vi "Actor Core.vi"(8 "error in":errorcluster, 11 "RandomDataChart in":refnum<class "ValueInputs.lvclass">) -> (0 "error out":errorcluster, 3 "Actor out":refnum<class "Actor.lvclass">)   [LabVIEW 2015, in "TestViewables.lvlib" / "ValueInputs.lvclass"]
doc: "(<B>Filename</B>: Actor Framework.lvlib:Actor.lvclass:Actor Core.vi)\n\nReceives messages to the actor, reacts to them, and initiates any error handling that may shut the actor down.\n\nDescendant classes may override this VI to append parallel tasks for the actor to complete while it handles messages. Overrides use the Call Parent Method node.\n\n<License>\nCopyright © 2017 Composed Systems, LLC | All rights reserved\nwww.composed.io\n\nAuthor: Ethan Stern <ethan.stern@composed.io>\n\nThis software is provided \"AS IS\" WITHOUT WARRANTIES, either express or implied, AND IS FOR EDUCATIONAL PURPOSES ONLY.\n</License>"
uses:
  ValueInputs.lvclass
  <vilib>/ActorFramework/Actor/Actor.lvclass
  <vilib>/ActorFramework/Actor/Actor.lvclass/Actor.ctl
  <vilib>/ActorFramework/Message Enqueuer/Message Enqueuer.lvclass/Message Enqueuer.ctl
  <vilib>/ActorFramework/Message Enqueuer/Init from Existing Queue.vi
  Framework/IViewable/IViewable/IViewable.lvclass
  <vilib>/ActorFramework/Message Enqueuer/Message Enqueuer.lvclass
  Framework/AutoRegistration/ActorAutoRegistration Messages/ValueChangeMsg/ValueChangeMsg.lvclass
panel:
  in  "ID":i32
  in  "Flavor":string
  in  "Setpoint":dbl
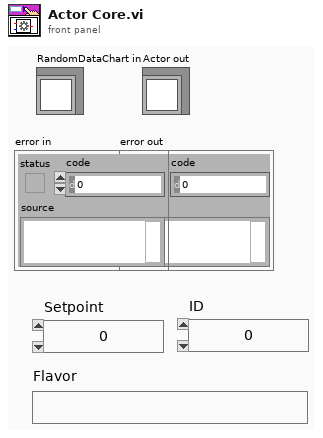
[diagram p1: front panel]
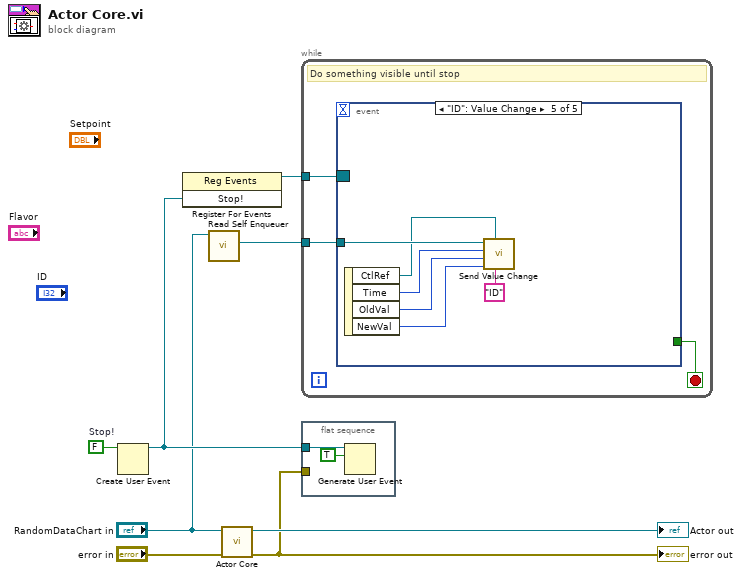
[diagram p0: block diagram]
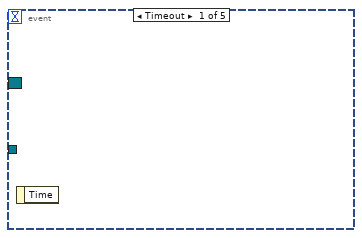
[diagram p2: hidden frame]
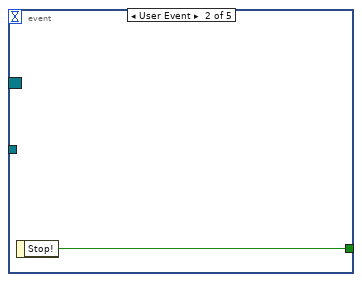
[diagram p3: hidden frame]
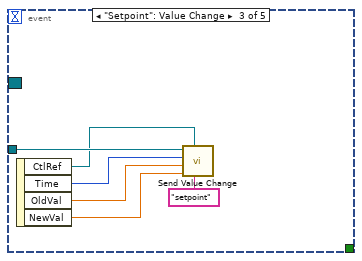
[diagram p4: hidden frame]
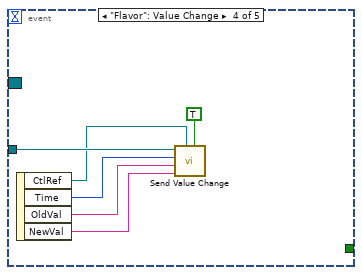
[diagram p5: hidden frame]
diagram:
  w6 = FALSE  # Stop!
  n1 = Create User Event(user event datatype=w6) -> (user event=w3:refnum<user-event>)  [unwired: 1 in, 1 out]
  n2 = register-events(w3) -> (reference out=w4:refnum<event-registration>)  [unwired: 2 in, 1 out]
  n3 = call <vilib>:"Read Self Enqueuer.vi"("Actor"="RandomDataChart in") -> ("Self Enqueuer"=w1:refnum<class "Message Enqueuer.lvclass">)  [unwired: 10 in]
  n4 = call-parent "Actor Core.vi"("error in"="error in", "IViewable In"="RandomDataChart in") -> ("error out"=w5:errorcluster, "Actor out"=→"Actor out":refnum<class "Actor.lvclass">)  [unwired: 8 in]
  "error out" <- w5
  n5 = while {
    tunnel: w4 -> [w11]
    tunnel: w1 -> [w9]
    stop <- w10 stop-if-true
    # "Do something visible until stop"
    n6 = event shown="[4] \"ID\": Value Change" {
      selector: w11 -> [_ _ _ _ _]
      dyn-events: _ -> [_ _ _ _ _]
      timeout: _ -> [_ _ _ _ _]
      tunnel: [_ w12 _ _ _] -> w10
      tunnel: w9 -> [_ _ w18 w24 w30]
      event Timeout {
        n7 = event-data() -> ()  [unwired: 1 in, 1 out]
      }
      event User Event {
        n8 = event-data() -> ("Stop!"=w12:bool)  [unwired: 1 in]
      }
      event "Setpoint": Value Change {
        n9 = event-data() -> ("CtlRef"=w13:refnum<vi>, "Time"=w14:u32, "OldVal"=w17:dbl, "NewVal"=w15:dbl)  [unwired: 1 in]
        n10 = call "Send Value Change.vi"("Name (Get Text From Control)"="setpoint" ("Name"), "Ctl Refnum"=w13, "New Value"=w15, "Old Value"=w17, "Time"=w14, "Message Enqueuer in"=w18) -> ()  [unwired: 5 in, 1 out]
      }
      event "Flavor": Value Change {
        n11 = event-data() -> ("CtlRef"=w23:refnum<vi>, "Time"=w22:u32, "OldVal"=w21:string, "NewVal"=w20:string)  [unwired: 1 in]
        n12 = call "Send Value Change.vi"("Use Label Text (F=Use Caption)"=TRUE, "Ctl Refnum"=w23, "New Value"=w20, "Old Value"=w21, "Time"=w22, "Message Enqueuer in"=w24) -> ()  [unwired: 5 in, 1 out]
      }
      event "ID": Value Change {
        n13 = event-data() -> ("CtlRef"=w27:refnum<vi>, "Time"=w26:u32, "OldVal"=w29:i32, "NewVal"=w25:i32)  [unwired: 1 in]
        n14 = call "Send Value Change.vi"("Name (Get Text From Control)"="ID" ("Name"), "Ctl Refnum"=w27, "New Value"=w25, "Old Value"=w29, "Time"=w26, "Message Enqueuer in"=w30) -> ()  [unwired: 5 in, 1 out]
      }
    }
  }
  n15 = flat-sequence {
    tunnel: w3 -> [w32]
    tunnel: w5 -> [_]
    frame #0 {
      n16 = Generate User Event(user event=w32, event data cluster=TRUE ("event data")) -> ()  [unwired: 2 in, 2 out]
    }
  }
